vi "Config Load2.vi"(8 "error in (no error)":errorcluster, 11 "Text":string) -> (0 "error out":errorcluster, 3 "skvc":string[][](array[string]))   [LabVIEW 2018]
uses:
  <vilib>/regexp/Match Regular Expression.xnode
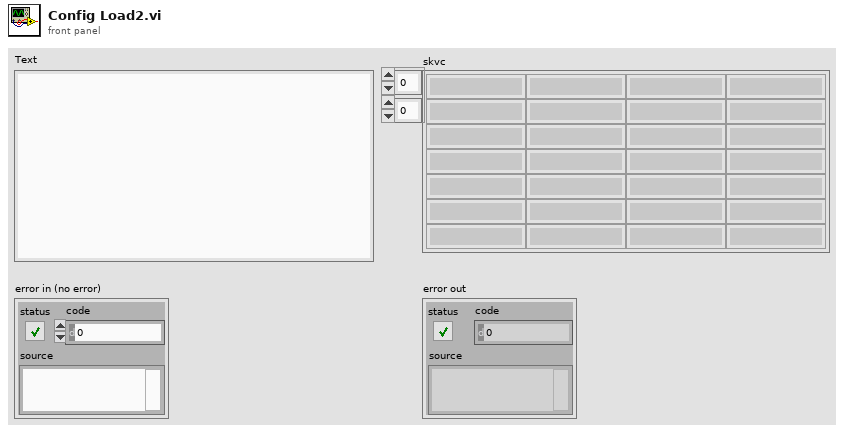
[diagram p1: front panel]
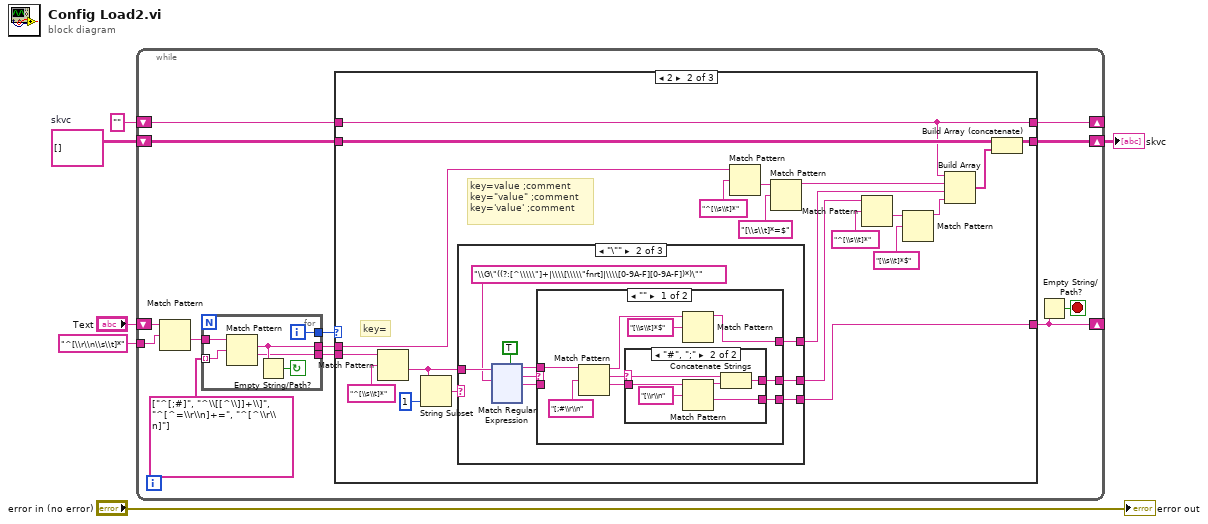
[diagram p0: block diagram]
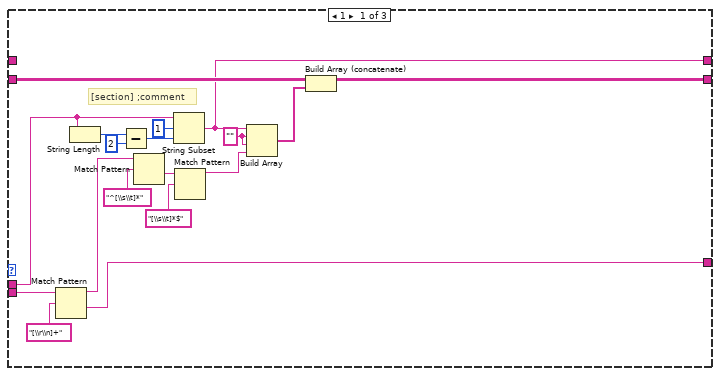
[diagram p2: hidden frame]
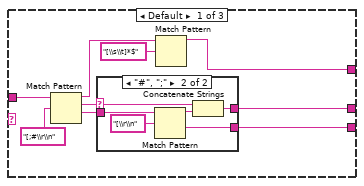
[diagram p3: hidden frame]
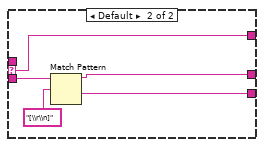
[diagram p6: hidden frame]
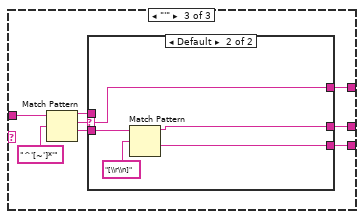
[diagram p7: hidden frame]
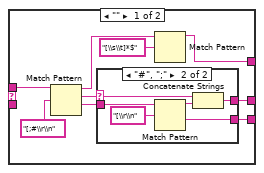
[diagram p8: hidden frame]
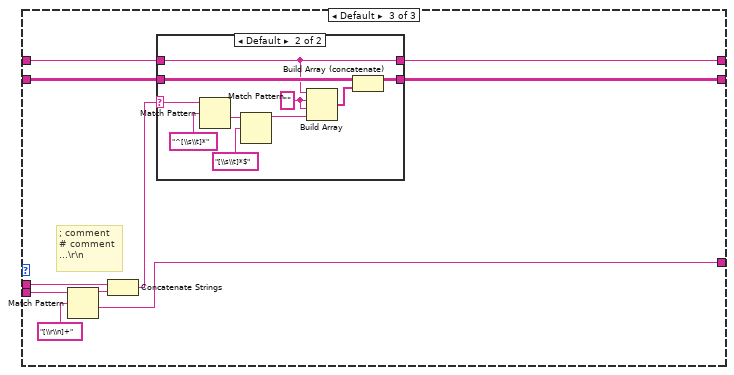
[diagram p10: hidden frame]
diagram:
  w2 = string[][] []  # skvc
  n1 = while {
    tunnel: "^[\\r\\n\\s\\t]*" ("regular expression") -> [w19]
    shift-right: [w12] -> _
    shift-left: "Text" -> [w18]
    shift-right: [w13] -> w1
    shift-left: w2 -> [w15]
    shift-right: [w7] -> _
    shift-left: "" ("Section") -> [w8]
    stop <- w11 stop-if-true
    n2 = Match Pattern(string=w18, regular expression=w19) -> (after substring=w17:string)  [unwired: 1 in, 3 out]
    n3 = for {
      tunnel: string[] ["^[;#]", "^\\[[^\\]]+\\]", "^[^=\\r\\n]+=", "^[^\\r\\n]"] -> [w278] mode=indexing
      tunnel: w17 -> [w277]
      tunnel: [w275] -> w10
      tunnel: [w274] -> w16
      tunnel: [w273] -> w14
      i -> [w274]
      stop <- w276 continue-if-true
      n4 = Match Pattern(string=w277, regular expression=w278) -> (match substring=w275:string, after substring=w273:string)  [unwired: 1 in, 2 out]
      n5 = Empty String/Path?(string/path=w275) -> (empty?=w276:bool)
    }
    n6 = case shown="2" w16 {
      tunnel: w15 -> [w28 w40 w260]
      tunnel: w14 -> [w25 w48 w256]
      tunnel: [w27 w39 w259] -> w13
      tunnel: [w24 w44 w255] -> w12
      tunnel: w10 -> [w26 w51 w253]
      tunnel: w8 -> [_ w38 w252]
      tunnel: [w23 w38 w251] -> w7
      frame 1 {
        w22 = ""
        # "[section] ;comment"
        n7 = Match Pattern(string=w25, regular expression="[\\r\\n]+") -> (before substring=w29:string, after substring=w24:string)  [unwired: 1 in, 2 out]
        n8 = String Length(string=w26) -> (length=w35:i32)
        n9 = Subtract(x=w35, y=2) -> (x-y=w33:i32)
        n10 = Match Pattern(string=w29, regular expression="^[\\s\\t]*") -> (after substring=w30:string)  [unwired: 1 in, 3 out]
        n11 = String Subset(string=w26, offset (0)=1, length (rest)=w33) -> (substring=w23:string)
        n12 = Match Pattern(string=w30, regular expression="[\\s\\t]*$") -> (before substring=w21:string)  [unwired: 1 in, 3 out]
        n13 = Build Array(w23, w22, w22, w21) -> (w20:string[])
        n14 = Build Array (concatenate)(w28, w20) -> (w27:string[][])
      }
      frame 2 {
        # "key=value ;comment\nkey=\"value\" ;comment\nkey='value' ;comment"
        # "key="
        n15 = Match Pattern(string=w48, regular expression="^[\\s\\t]*") -> (after substring=w45:string)  [unwired: 1 in, 3 out]
        n16 = String Subset(string=w45, length (rest)=1 ("length (rest)")) -> (substring=w46:string)  [unwired: 1 in]
        n17 = case shown="\"\\\"\"" w46 {
          tunnel: w45 -> [w66 w83 w226]
          tunnel: [w63 w76 w227] -> w44
          tunnel: [w62 w77 w228] -> w43
          tunnel: [w59 w80 w229] -> w42
          frame Default {
            n18 = Match Pattern(string=w66, regular expression="[;#\\r\\n") -> (before substring=w60:string, match substring=w64:string, after substring=w65:string)  [unwired: 1 in, 1 out]
            n19 = case shown="\"#\", \";\"" w64 {
              selector: w64 -> [_ w72]
              tunnel: w65 -> [w68 w73]
              tunnel: [w68 w70] -> w63
              tunnel: [_ w69] -> w62
              frame Default {
              }
              frame "#", ";" {
                n20 = Match Pattern(string=w73, regular expression="[\\r\\n") -> (before substring=w71:string, after substring=w70:string)  [unwired: 1 in, 2 out]
                n21 = Concatenate Strings(w72, w71) -> (w69:string)
              }
            }
            n22 = Match Pattern(string=w60, regular expression="[\\s\\t]*$") -> (before substring=w59:string)  [unwired: 1 in, 3 out]
          }
          frame "\"" {
            n23 = xnode "Match Regular Expression"("input string"=w83, "regular expression"="\\G\"((?:[^\\\\\"]+|\\\\[\\\\\"fnrt]|\\\\[0-9A-F][0-9A-F])*)\"", "multiline? (F)"=TRUE) -> ("before match"=w79:string, "whole match"=w81:string, "after match"=w78:string)  [unwired: 3 in, 2 out]
            n24 = case shown="\"\"" w81 {
              selector: w81 -> [_ w104]
              tunnel: [w84 w104] -> w80
              tunnel: w79 -> [w89 _]
              tunnel: w78 -> [_ w102]
              tunnel: [w88 w101] -> w77
              tunnel: [w87 w100] -> w76
              frame "" {
                n25 = Match Pattern(string=w89, regular expression="[;#\\r\\n") -> (before substring=w85:string, match substring=w90:string, after substring=w91:string)  [unwired: 1 in, 1 out]
                n26 = case shown="\"#\", \";\"" w90 {
                  selector: w90 -> [_ w97]
                  tunnel: w91 -> [w93 w98]
                  tunnel: [w93 w95] -> w87
                  tunnel: [_ w94] -> w88
                  frame Default {
                  }
                  frame "#", ";" {
                    n27 = Match Pattern(string=w98, regular expression="[\\r\\n") -> (before substring=w96:string, after substring=w95:string)  [unwired: 1 in, 2 out]
                    n28 = Concatenate Strings(w97, w96) -> (w94:string)
                  }
                }
                n29 = Match Pattern(string=w85, regular expression="[\\s\\t]*$") -> (before substring=w84:string)  [unwired: 1 in, 3 out]
              }
              frame Default {
                n30 = Match Pattern(string=w102, regular expression="[\\r\\n]") -> (before substring=w101:string, after substring=w100:string)  [unwired: 1 in, 2 out]
              }
            }
          }
          frame "'" {
            n31 = Match Pattern(string=w226, regular expression="^'[~']*'") -> (before substring=w225:string, match substring=w224:string, after substring=w223:string)  [unwired: 1 in, 1 out]
            n32 = case shown="Default" w224 {
              selector: w224 -> [_ w250]
              tunnel: [w230 w250] -> w229
              tunnel: w225 -> [w235 _]
              tunnel: w223 -> [_ w248]
              tunnel: [w234 w247] -> w228
              tunnel: [w233 w246] -> w227
              frame "" {
                n33 = Match Pattern(string=w235, regular expression="[;#\\r\\n") -> (before substring=w231:string, match substring=w236:string, after substring=w237:string)  [unwired: 1 in, 1 out]
                n34 = case shown="\"#\", \";\"" w236 {
                  selector: w236 -> [_ w243]
                  tunnel: w237 -> [w239 w244]
                  tunnel: [w239 w241] -> w233
                  tunnel: [_ w240] -> w234
                  frame Default {
                  }
                  frame "#", ";" {
                    n35 = Match Pattern(string=w244, regular expression="[\\r\\n") -> (before substring=w242:string, after substring=w241:string)  [unwired: 1 in, 2 out]
                    n36 = Concatenate Strings(w243, w242) -> (w240:string)
                  }
                }
                n37 = Match Pattern(string=w231, regular expression="[\\s\\t]*$") -> (before substring=w230:string)  [unwired: 1 in, 3 out]
              }
              frame Default {
                n38 = Match Pattern(string=w248, regular expression="[\\r\\n]") -> (before substring=w247:string, after substring=w246:string)  [unwired: 1 in, 2 out]
              }
            }
          }
        }
        n39 = Match Pattern(string=w51, regular expression="^[\\s\\t]*") -> (after substring=w54:string)  [unwired: 1 in, 3 out]
        n40 = Match Pattern(string=w54, regular expression="[\\s\\t]*=$") -> (before substring=w50:string)  [unwired: 1 in, 3 out]
        n41 = Match Pattern(string=w43, regular expression="^[\\s\\t]*") -> (after substring=w56:string)  [unwired: 1 in, 3 out]
        n42 = Match Pattern(string=w56, regular expression="[\\s\\t]*$") -> (before substring=w55:string)  [unwired: 1 in, 3 out]
        n43 = Build Array(w38, w50, w42, w55) -> (w41:string[])
        n44 = Build Array (concatenate)(w40, w41) -> (w39:string[][])
      }
      frame Default {
        # "; comment\n# comment\n...\\r\\n"
        n45 = Match Pattern(string=w256, regular expression="[\\r\\n]+") -> (before substring=w257:string, after substring=w255:string)  [unwired: 1 in, 2 out]
        n46 = Concatenate Strings(w253, w257) -> (w254:string)
        n47 = case shown="Default" w254 {
          selector: w254 -> [_ w268]
          tunnel: w260 -> [w262 w264]
          tunnel: [w262 w265] -> w259
          tunnel: w252 -> [w261 w263]
          tunnel: [w261 w263] -> w251
          frame "" {
          }
          frame Default {
            w267 = ""
            n48 = Match Pattern(string=w268, regular expression="^[\\s\\t]*") -> (after substring=w270:string)  [unwired: 1 in, 3 out]
            n49 = Match Pattern(string=w270, regular expression="[\\s\\t]*$") -> (before substring=w269:string)  [unwired: 1 in, 3 out]
            n50 = Build Array(w263, w267, w267, w269) -> (w266:string[])
            n51 = Build Array (concatenate)(w264, w266) -> (w265:string[][])
          }
        }
      }
    }
    n52 = Empty String/Path?(string/path=w12) -> (empty?=w11:bool)
  }
  "skvc" <- w1
  "error out" <- "error in (no error)"
